vi "Contour Line_Interpolation Contour Point.vi"(5 "z 2":dbl, 6 "height":dbl, 7 "z 1":dbl, 8 "y 2":dbl, 9 "y 1":dbl, 10 "x 2":dbl, 11 "x 1":dbl) -> (3 "contour point":cluster{"x":dbl, "y":dbl})   [LabVIEW 2020, in "NI_AAL_Geometry.lvlib"]
uses:
  <vilib>/Analysis/NI_AAL_Geometry.lvlib
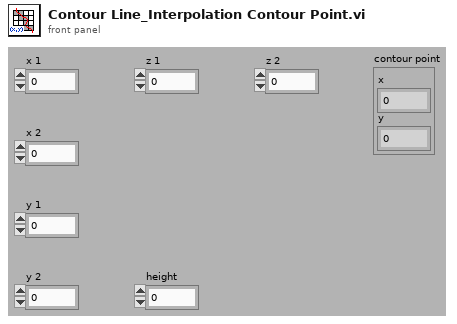
[diagram p1: front panel]
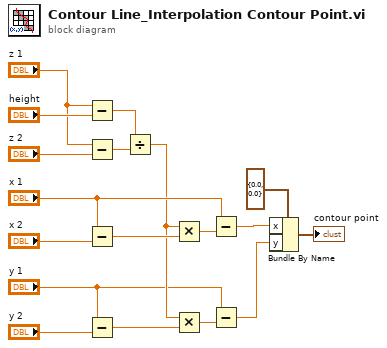
[diagram p0: block diagram]
diagram:
  n1 = Subtract(x="z 1", y="height") -> (x-y=w15:dbl)
  n2 = Subtract(x="z 1", y="z 2") -> (x-y=w14:dbl)
  n3 = Subtract(x="x 1", y="x 2") -> (x-y=w12:dbl)
  n4 = Subtract(x="y 1", y="y 2") -> (x-y=w8:dbl)
  n5 = Divide(x=w15, y=w14) -> (x/y=w6:dbl)
  n6 = Multiply(x=w6, y=w12) -> (x*y=w10:dbl)
  n7 = Multiply(x=w6, y=w8) -> (x*y=w9:dbl)
  n8 = Subtract(x="x 1", y=w10) -> (x-y=w5:dbl)
  n9 = Subtract(x="y 1", y=w9) -> (x-y=w3:dbl)
  n10 = Bundle By Name(cluster=cluster{"x":dbl, "y":dbl} {"x"=0.0, "y"=0.0} ("contour point 2"), "x"=w5, "y"=w3) -> (→"contour point":cluster{"x":dbl, "y":dbl})
